vi "Save Results to TDMS.vi"(8 "error in (no error)":errorcluster, 10 "measurement configuration":T1={"Mode of operation"=enum."Perform measurement", "DUT setup time"=1.0, "Source delay"=0.005, "Aperture time"=0.005, "Nominal output voltage"=3.3, "Source pin name array"=[], "Source pin name index for efficiency"=0, "Source sense array"=[], "Source current limit array"=[], "Source maximum power array"=[], "Source start voltage array"=[], "Source stop voltage array"=[], "Source voltage sweep points"=4, "Use Source voltage array"=FALSE, "Source voltage concatenated array"=[], "Source voltage array size"=[], "Load pin name"="", "Load sense"=1009, "Load voltage limit range"=6.0, "Load sweep type"="Logarithmic", "Load start current"=0.1, "Load stop current"=24.0, "Load current sweep points/points per decade"=10, "Use Load current array"=FALSE, "Load current array"=[], "Pin Names for Scope"=[], "vertical range"=[], "vertical offset"=[], "probe attenuation"=[], "vertical coupling"=[], "channel enabled"=[], "input impedance"=[], "max input frequency"=[], "min sample rate"=[], "reference position"=[], "min record length"=[], "enforce realtime"=[], "dmm pin names"=[], "dmm function array"=[], "dmm resolution in digits array"=[], "dmm range array"=[]} {"dmm function array" items=["DC Volts", "AC Volts", "DC Current", "AC Current", "2-wire Resistance", "4-wire Resistance", "Diode", "Frequency", "Period", "AC Volts DC Coupled", "Capacitance", "Inductance", "Temperature"]; "Source sense array" items=["Local"=1008, "Remote"=1009]; "dmm resolution in digits array" items=["3 1/2"=3.5, "4 1/2"=4.5, "5 1/2"=5.5, "6 1/2"=6.5, "7 1/2"=7.5]; "input impedance" items=["1 mega ohm"=0, "50 ohms"=2]; "vertical coupling" items=["AC", "DC", "Ground"]; "Load sense" items=["Local"=1008, "Remote"=1009]}, 11 "Reference values":T4={"dcpower session reservation"=refnum, "Source handle array"=[], "Source channel name array"=[], "Load handle"="", "Load channel name"="", "Source voltage values"=[], "Load current values"=[], "Number of steps"=0, "Source sequence name"="", "Source terminal name"="", "Measure terminal name"="", "scope session reservation"=refnum, "Scope handles"=[], "connection map"={}, "instrument info map array"=[], "Enable TClk"=FALSE, "dmm session reservation"=refnum, "dmm handle array"=[], "DMM Trigger Source"=enum."Immediate", "DMM Sample Trigger"=enum."TTL 0", "Measurement Results"={"Status"="", "Voltage values"=[], "Source sweep points"=0, "Load sweep points"=0, "Source voltages"=[], "Source currents"=[], "Load voltages"=[], "Load currents"=[], "Load voltage deviation"=[], "Efficiency"=[], "Maximum efficiency"=[], "Minimum load voltage"=[], "Maximum load voltage"=[], "Minimum load regulation"=[], "Maximum load regulation"=[], "waveform pins"=[], "waveform sites"=[], "waveform t0 array"=[], "waveform dt array"=[], "waveform length array"=[], "concatenated waveform Y"=[]}, "Additional measurements"={"voltage measurements from all sources"=[], "current measurements from all sources"=[], "all dmm measurements"=[], "all scope waverforms"=[]}}) -> (0 "error out":errorcluster)   [LabVIEW 2021, in "Efficiency And Load Regulation with Pin Map.lvlib"]
uses:
  Efficiency And Load Regulation with Pin Map.lvlib
  Reference values.ctl
  <vilib>/Plug-In SDKs/Clients/Session Management V1/Session Reservation/Session Reservation.lvclass
  common/Instrument Control/Scope/TClk/Instrument Info.ctl
  common/Instrument Control/Scope Parameters.ctl
  <instrlib>/niScope/Controls/niScope vertical coupling.ctl
  <instrlib>/niDMM/nidmm.llb/niDMM Trigger.ctl
  <instrlib>/niDMM/nidmm.llb/niDMM Sample Trigger.ctl
  Measurement Results.ctl
  Additional measurements.ctl
  Measurement Configuration.ctl
  <instrlib>/niDMM/nidmm.llb/niDMM Resolution in Digits.ctl
  <vilib>/Utility/sysdir.llb/System Directory Type.ctl
  common/PMIC Common.lvlib
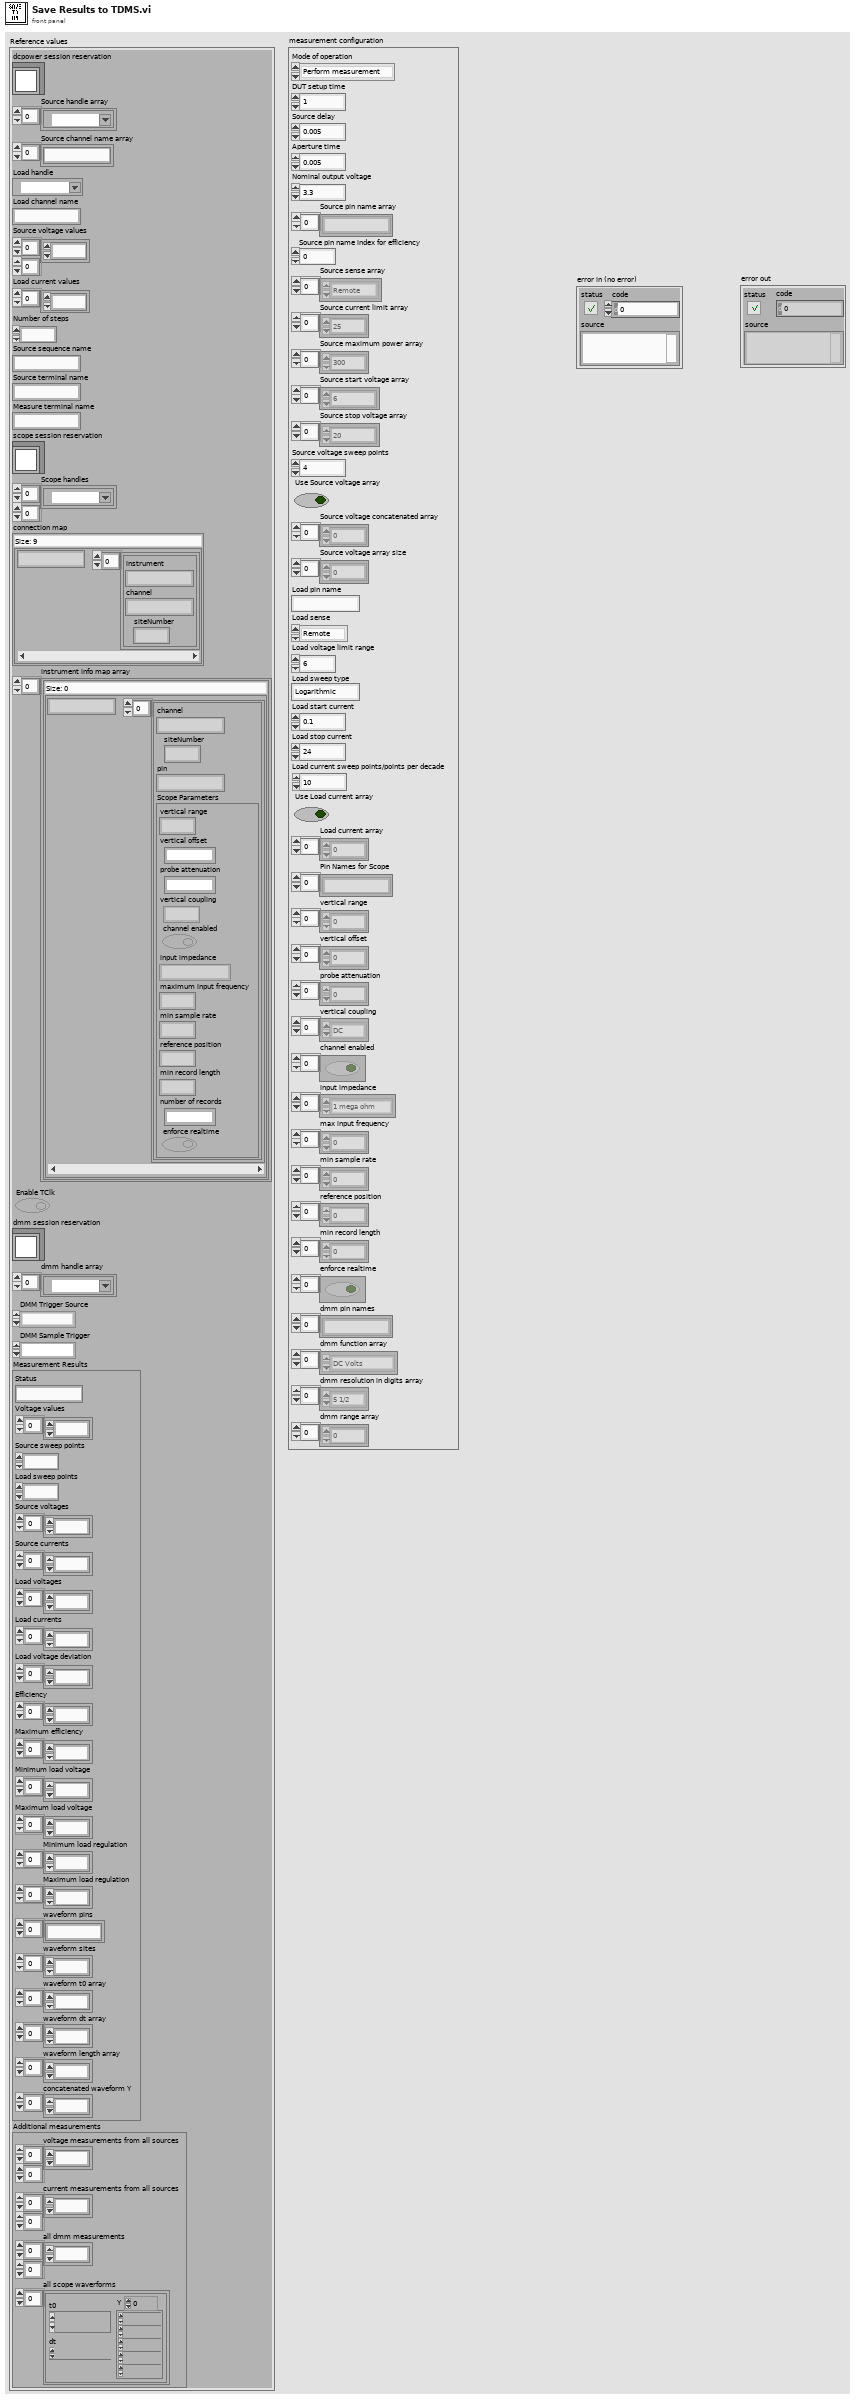
[diagram p1: front panel]
types:
  T1 = typedef "Efficiency And Load Regulation with Pin Map.lvlib/Measurement Configuration.ctl" = cluster{"Mode of operation":enum32{"Power on the DUT", "Perform measurement", "Power off the DUT"}, "DUT setup time":dbl, "Source delay":dbl, "Aperture time":dbl, "Nominal output voltage":dbl, "Source pin name array":string[], "Source pin name index for efficiency":i32, "Source sense array":i32[], "Source current limit array":dbl[], "Source maximum power array":dbl[], "Source start voltage array":dbl[], "Source stop voltage array":dbl[], "Source voltage sweep points":i32, "Use Source voltage array":bool, "Source voltage concatenated array":dbl[], "Source voltage array size":i32[], "Load pin name":string, "Load sense":i32, "Load voltage limit range":dbl, "Load sweep type":string, "Load start current":dbl, "Load stop current":dbl, "Load current sweep points/points per decade":i32, "Use Load current array":bool, "Load current array":dbl[], "Pin Names for Scope":string[], "vertical range":dbl[], "vertical offset":dbl[], "probe attenuation":dbl[], "vertical coupling":T2[], "channel enabled":bool[], "input impedance":u32[], "max input frequency":dbl[], "min sample rate":dbl[], "reference position":dbl[], "min record length":i32[], "enforce realtime":bool[], "dmm pin names":string[], "dmm function array":u32[], "dmm resolution in digits array":T3[], "dmm range array":dbl[]}
  T2 = typedef "niScope vertical coupling.ctl" = i32
  T3 = typedef "niDMM Resolution in Digits.ctl" = dbl
  T4 = typedef "Efficiency And Load Regulation with Pin Map.lvlib/Reference values.ctl" = cluster{"dcpower session reservation":refnum<class "Session Reservation.lvclass">, "Source handle array":refnum<k15>[], "Source channel name array":string[], "Load handle":refnum<k15>, "Load channel name":string, "Source voltage values":dbl[][], "Load current values":dbl[], "Number of steps":i32, "Source sequence name":string, "Source terminal name":string, "Measure terminal name":string, "scope session reservation":refnum<class "Session Reservation.lvclass">, "Scope handles":refnum<k15>[][], "connection map":map{string, T5[]}, "instrument info map array":map{string, cluster{"channel":string, "siteNumber":i32, "pin":string, "Scope Parameters":T6}[]}[], "Enable TClk":bool, "dmm session reservation":refnum<class "Session Reservation.lvclass">, "dmm handle array":refnum<k15>[], "DMM Trigger Source":T7, "DMM Sample Trigger":T8, "Measurement Results":T9, "Additional measurements":T10}
  T5 = typedef "PMIC Common.lvlib/Instrument Info.ctl" = cluster{"instrument":string, "channel":string, "siteNumber":i32}
  T6 = typedef "PMIC Common.lvlib/Scope Parameters.ctl" = cluster{"vertical range":dbl, "vertical offset":dbl, "probe attenuation":dbl, "vertical coupling":T2, "channel enabled":bool, "input impedance":u32, "maximum input frequency":dbl, "min sample rate":dbl, "reference position":dbl, "min record length":i32, "number of records":i32, "enforce realtime":bool}
  T7 = typedef "niDMM Trigger.ctl" = enum16{"Immediate", "External", "TTL 0", "TTL 1", "TTL 2", "TTL 3", "TTL 4", "TTL 5", "TTL 6", "Software", "TTL 7", "PXI Star", "LBR Trig 1", "Aux Trig 1"}
  T8 = typedef "niDMM Sample Trigger.ctl" = enum16{"Immediate", "External", "TTL 0", "TTL 1", "TTL 2", "TTL 3", "TTL 4", "TTL 5", "TTL 6", "Interval", "Software", "TTL 7", "PXI Star", "LBR Trig 1", "Aux Trig 1"}
  T9 = typedef "Efficiency And Load Regulation with Pin Map.lvlib/Measurement Results.ctl" = cluster{"Status":string, "Voltage values":dbl[], "Source sweep points":i32, "Load sweep points":i32, "Source voltages":dbl[], "Source currents":dbl[], "Load voltages":dbl[], "Load currents":dbl[], "Load voltage deviation":dbl[], "Efficiency":dbl[], "Maximum efficiency":dbl[], "Minimum load voltage":dbl[], "Maximum load voltage":dbl[], "Minimum load regulation":dbl[], "Maximum load regulation":dbl[], "waveform pins":string[], "waveform sites":i32[], "waveform t0 array":dbl[], "waveform dt array":dbl[], "waveform length array":i32[], "concatenated waveform Y":dbl[]}
  T10 = typedef "Efficiency And Load Regulation with Pin Map.lvlib/Additional measurements.ctl" = cluster{"voltage measurements from all sources":dbl[][], "current measurements from all sources":dbl[][], "all dmm measurements":dbl[][], "all scope waverforms":waveform(dbl)[]}
  T11 = typedef "System Directory Type.ctl" = i32
  T12 = enum16{"open", "open or create", "create or replace", "create", "open (read-only)"}
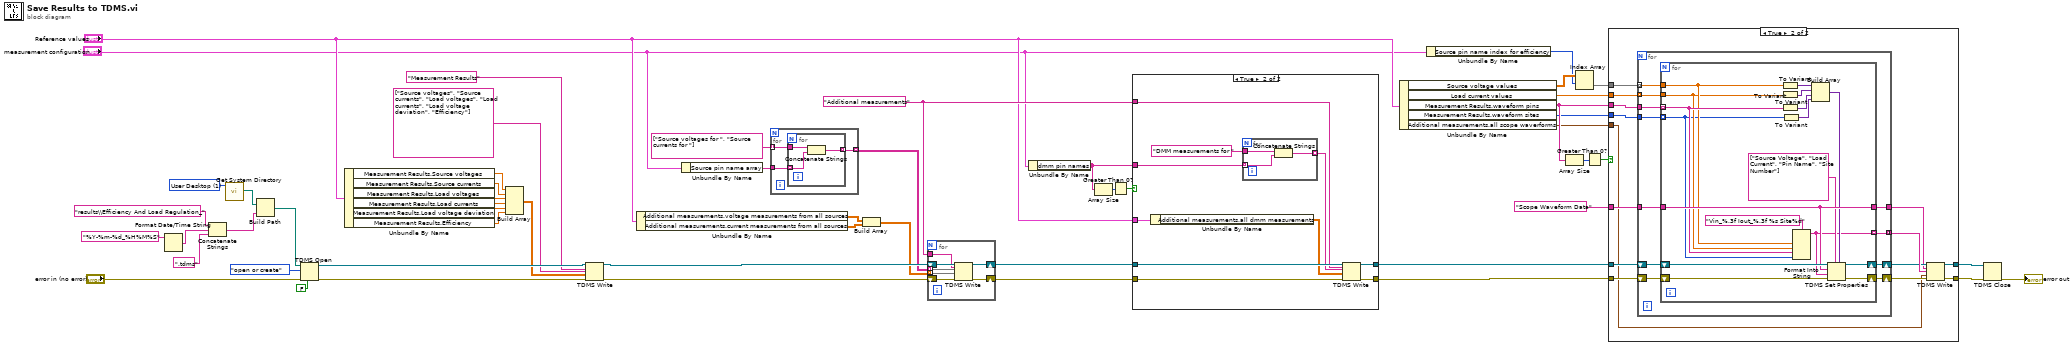
[diagram p0: block diagram]
diagram:
  w17 = "Additional measurements" ("group name in (Untitled)")
  w34 = T11 1 items=["User Home"=0, "User Desktop"=1, "User Documents"=2, "User Application Data"=3, "User Preferences"=4, "User Temporary"=5, "Public Documents"=6, "Public Application Data"=7, "Public Preferences"=8, "Public Cache"=13, "System Core Libraries"=9, "System Installed Libraries"=10, "Application Files"=11, "Boot Volume Root"=12] ("system directory type")
  n1 = Format Date/Time String(time format string (%c)="%Y-%m-%d_%H%M%S") -> (date/time string=w4:string)  [unwired: 2 in]
  n2 = Concatenate Strings("results\\Efficiency And Load Regulation_", w4, ".tdms" ("string")) -> (w1:string)
  n3 = call <vilib>:"Get System Directory.vi"("system directory type"=w34) -> ("system directory"=w33:path)  [unwired: 10 in]
  n4 = Build Path(base path=w33, name or relative path=w1) -> (appended path=w45:path)
  n5 = TDMS Open(6:FALSE ("disable buffering? (T)"), 8:"error in (no error)", 10:T12."open or create" ("operation (0:open)"), 11:w45) -> (0:w43:errorcluster, 3:w44:refnum<k34>)  [unwired: 3 in]
  n6 = Unbundle By Name("Reference values") -> ("Measurement Results.Source voltages"=w42:dbl[], "Measurement Results.Source currents"=w41:dbl[], "Measurement Results.Load voltages"=w40:dbl[], "Measurement Results.Load currents"=w39:dbl[], "Measurement Results.Load voltage deviation"=w38:dbl[], "Measurement Results.Efficiency"=w37:dbl[])
  n7 = Build Array(w42, w41, w40, w39, w38, w37) -> (w36:dbl[][])
  n8 = TDMS Write(0:w44, 5:"Measurement Results" ("group name in (Untitled)"), 7:string[] ["Source voltages", "Source currents", "Load voltages", "Load currents", "Load voltage deviation", "Efficiency"], 9:w36, 11:w43) -> (4:w25:refnum<k34>, 15:w26:errorcluster)  [unwired: 1 in, 2 out]
  n9 = Unbundle By Name("Reference values") -> ("Additional measurements.voltage measurements from all sources"=w29:dbl[][], "Additional measurements.current measurements from all sources"=w28:dbl[][])
  n10 = Unbundle By Name("measurement configuration") -> ("Source pin name array"=w23:string[])
  n11 = for {
    tunnel: w23 -> [w56]
    tunnel: string[] ["Source voltages for ", "Source currents for "] -> [w55] mode=indexing
    tunnel: [w54] -> w16 mode=indexing
    n12 = for {
      tunnel: w56 -> [w58] mode=indexing
      tunnel: w55 -> [w59]
      tunnel: [w57] -> w54 mode=indexing
      n13 = Concatenate Strings(w59, w58) -> (w57:string)
    }
  }
  n14 = Build Array(w29, w28) -> (w24:dbl[][][])
  n15 = for {
    shift-right: [w63] -> w21
    shift-left: w26 -> [w66]
    shift-right: [w64] -> w18
    shift-left: w25 -> [w65]
    tunnel: w17 -> [w62]
    tunnel: w16 -> [w60] mode=indexing
    tunnel: w24 -> [w61] mode=indexing
    n16 = TDMS Write(0:w65, 5:w62, 7:w60, 9:w61, 11:w66) -> (4:w64:refnum<k34>, 15:w63:errorcluster)  [unwired: 1 in, 2 out]
  }
  n17 = Unbundle By Name("measurement configuration") -> ("dmm pin names"=w14:string[])
  n18 = Array Size(array=w14) -> (size(s)=w12:i32)
  n19 = Greater Than 0?(x=w12) -> (x > 0?=w13:bool)
  n20 = case shown="True" w13 {
    tunnel: w14 -> [_ w77]
    tunnel: w21 -> [w68 w76]
    tunnel: [w68 w75] -> w20
    tunnel: [w67 w74] -> w19
    tunnel: w18 -> [w67 w73]
    tunnel: w17 -> [_ w72]
    tunnel: "Reference values" -> [_ w70]
    frame False {
    }
    frame True {
      n21 = Unbundle By Name(w70) -> ("Additional measurements.all dmm measurements"=w69:dbl[][])
      n22 = for {
        tunnel: "DMM measurements for " -> [w81]
        tunnel: w77 -> [w80] mode=indexing
        tunnel: [w79] -> w71 mode=indexing
        n23 = Concatenate Strings(w81, w80) -> (w79:string)
      }
      n24 = TDMS Write(0:w73, 5:w72, 7:w71, 9:w69, 11:w76) -> (4:w74:refnum<k34>, 15:w75:errorcluster)  [unwired: 1 in, 2 out]
    }
  }
  n25 = Unbundle By Name("Reference values") -> ("Source voltage values"=w8:dbl[][], "Load current values"=w51:dbl[], "Measurement Results.waveform pins"=w32:string[], "Measurement Results.waveform sites"=w31:i32[], "Additional measurements.all scope waverforms"=w30:waveform(dbl)[])
  n26 = Unbundle By Name("measurement configuration") -> ("Source pin name index for efficiency"=w7:i32)
  n27 = Array Size(array=w32) -> (size(s)=w11:i32)
  n28 = Index Array(array=w8, index (row)=w7) -> (element=w6:dbl[])  [unwired: 1 in]
  n29 = Greater Than 0?(x=w11) -> (x > 0?=w10:bool)
  n30 = case shown="True" w10 {
    tunnel: w51 -> [_ w97]
    tunnel: w32 -> [_ w95]
    tunnel: "Scope Waveform Data" ("group name in (Untitled)") -> [_ w92]
    tunnel: w6 -> [_ w90]
    tunnel: w20 -> [w83 w89]
    tunnel: w19 -> [w82 w88]
    tunnel: [w83 w87] -> w47
    tunnel: [w82 w86] -> w46
    tunnel: w31 -> [_ w85]
    tunnel: w30 -> [_ w84]
    frame False {
      # "Do nothing if Pin Names are emply."
    }
    frame True {
      n31 = for {
        tunnel: w95 -> [w106]
        tunnel: w90 -> [w108] mode=indexing
        tunnel: w97 -> [w107] mode=indexing
        tunnel: [w105] -> w96 mode=concatenating
        shift-right: [w104] -> w94
        shift-left: w88 -> [w99]
        shift-right: [w102] -> w93
        shift-left: w89 -> [w103]
        tunnel: w92 -> [w101]
        tunnel: [w100] -> w91
        tunnel: w85 -> [w98]
        n32 = for {
          tunnel: w108 -> [w117]
          tunnel: w107 -> [w116]
          tunnel: w106 -> [w118] mode=indexing
          tunnel: [w112] -> w105 mode=indexing
          shift-right: [w123] -> w104
          shift-left: w99 -> [w124]
          shift-right: [w121] -> w102
          shift-left: w103 -> [w122]
          tunnel: w101 -> [w120]
          tunnel: [w120] -> w100
          tunnel: w98 -> [w109] mode=indexing
          n33 = To Variant(anything=w117) -> (Variant=w115:variant)
          n34 = To Variant(anything=w116) -> (Variant=w114:variant)
          n35 = To Variant(anything=w118) -> (Variant=w111:variant)
          n36 = To Variant(anything=w109) -> (Variant=w110:variant)
          n37 = Format Into String(format string="Vin_%.3f Iout_%.3f %s Site%d", w117, w116, w118, w109) -> (resulting string=w112:string)  [unwired: 2 in, 1 out]
          n38 = Build Array(w115, w114, w111, w110) -> (w113:variant[])
          n39 = TDMS Set Properties(5:w113, 7:string[] ["Source Voltage", "Load Current", "Pin Name", "Site Number"] ("property names"), 8:w122, 9:w112, 10:w120, 11:w124) -> (0:w121:errorcluster, 3:w123:refnum<k34>)  [unwired: 2 out]
        }
      }
      n40 = TDMS Write(0:w94, 5:w91, 7:w96, 9:w84, 11:w93) -> (4:w86:refnum<k34>, 15:w87:errorcluster)  [unwired: 1 in, 2 out]
    }
  }
  n41 = TDMS Close(8:w47, 11:w46) -> (0:→"error out":errorcluster)  [unwired: 1 out]
